vi "Default Property or Method.vi"(8 "error in":errorcluster, 10 "Properties for Tree In":T1(array[cluster]), 11 "Affected Items":T2) -> (0 "error out":errorcluster, 3 "One default element":bool)   [LabVIEW 2023]
doc: "Determine if the property or invoke node contains only the default property (such as when the node is first dropped)."
uses:
  top/BundleMagic.ctl
panel:
  # "Take either input"
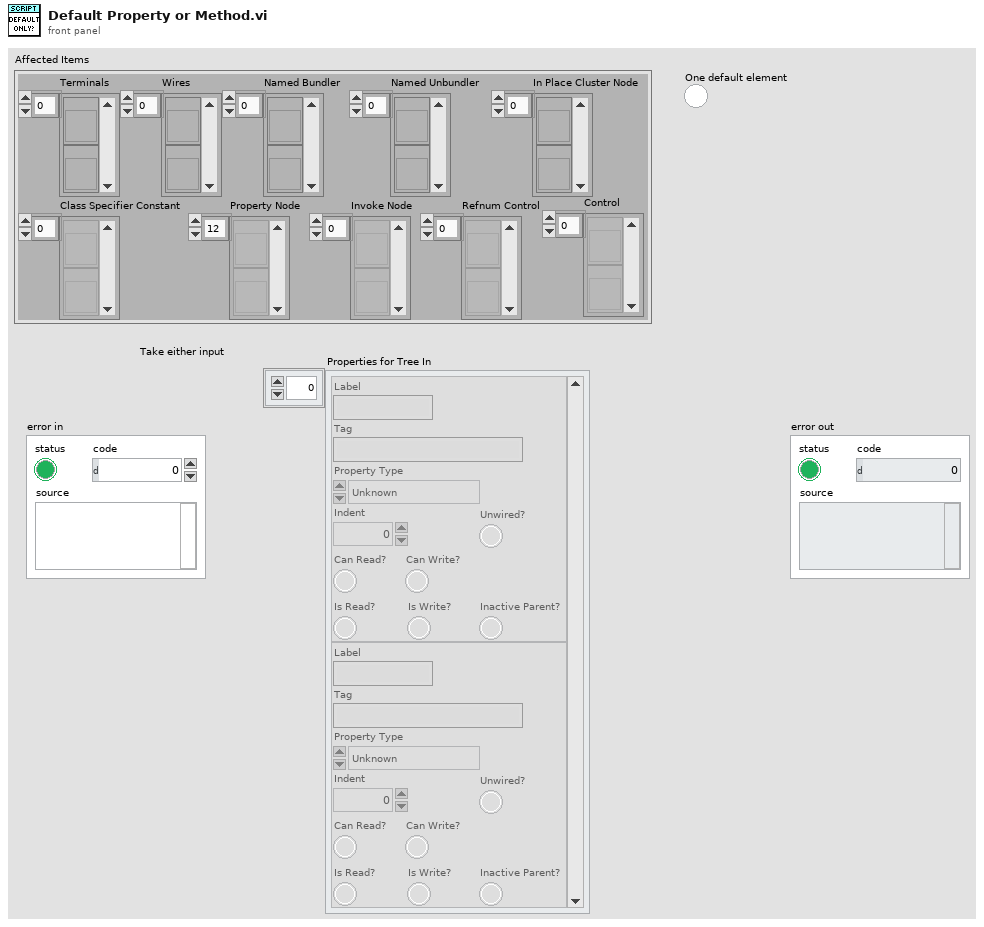
[diagram p1: front panel]
types:
  T1 = cluster{"Label":string, "Tag":string, "Property Type":enum16{"Unknown", "Base", "Scripting", "Private", "Deprecated", "None", "Divider"}, "Indent":u16, "Can Read?":bool, "Can Write?":bool, "Is Read?":bool, "Is Write?":bool, "Inactive Parent?":bool, "Unwired?":bool}[]
  T2 = typedef "BundleMagic.ctl" = cluster{"Terminals":refnum<vi>[], "Wires":refnum<vi>[], "Named Bundler":refnum<vi>[], "Named Unbundler":refnum<vi>[], "In Place Cluster Node":refnum<vi>[], "Class Specifier Constant":refnum<vi>[], "Property Node":refnum<vi>[], "Invoke Node":refnum<vi>[], "Refnum Control":refnum<vi>[], "Control":refnum<vi>[]}
  T3 = cluster{"Label":string, "Tag":string, "Property Type":enum16{"Unknown", "Base", "Scripting", "Private", "Deprecated", "None", "Divider"}, "Indent":u16, "Can Read?":bool, "Can Write?":bool, "Is Read?":bool, "Is Write?":bool, "Inactive Parent?":bool, "Unwired?":bool}
  T4 = typedef "ASPM_UniqueIDStringDatanameShortnameLongname.ctl" = cluster{"Unique ID string":string, "Data name":string, "Short name (localized)":string, "Long name (localized)":string}
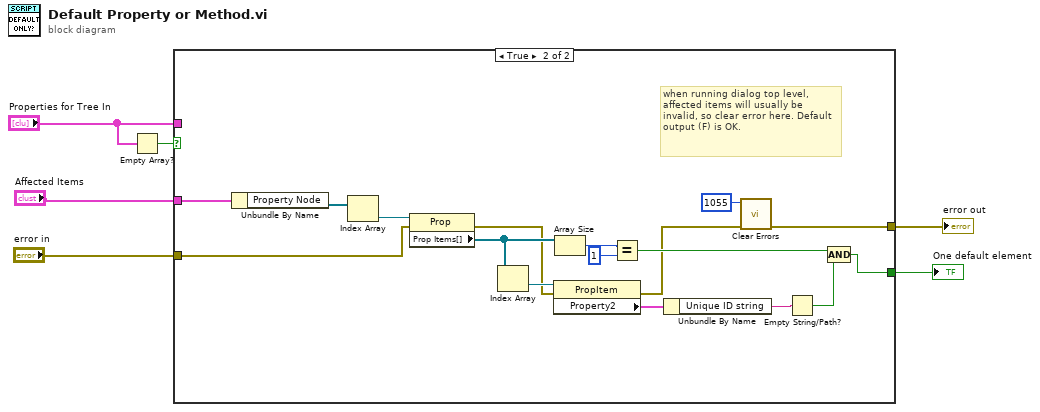
[diagram p0: block diagram]
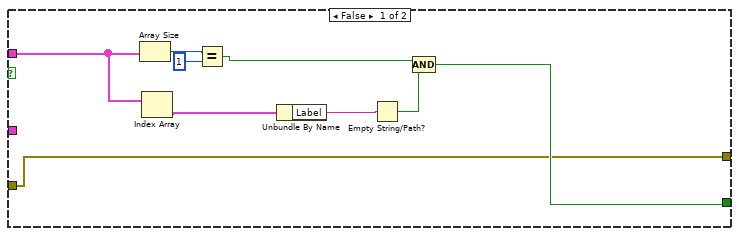
[diagram p2: hidden frame]
diagram:
  n1 = Empty Array?(array="Properties for Tree In") -> (empty?=w2:bool)
  n2 = case shown="True" w2 {
    tunnel: "Affected Items" -> [_ w31]
    tunnel: "error in" -> [w7 w30]
    tunnel: [w7 w17] -> w4
    tunnel: [w8 w29] -> w3
    tunnel: "Properties for Tree In" -> [w10 _]
    frame False {
      n3 = Array Size(array=w10) -> (size(s)=w15:i32)
      n4 = Index Array(array=w10) -> (element=w9:T3)  [unwired: 1 in]
      n5 = Equal?(x=w15, y=1) -> (x = y?=w14:bool)
      n6 = Unbundle By Name(w9) -> ("Label"=w13:string)
      n7 = Empty String/Path?(string/path=w13) -> (empty?=w12:bool)
      n8 = Compound Arithmetic op=AND(w14, w12) -> (w8:bool)
    }
    frame True {
      # "when running dialog top level, affected items will usually be invalid, so clear error here. Default output (F) is OK."
      n9 = Unbundle By Name(w31) -> ("Property Node"=w28:refnum<vi>[])
      n10 = Index Array(array=w28) -> (element=w32:refnum<vi>)  [unwired: 1 in]
      n11 = property class="Prop"(reference=w32, error in=w30) -> (error out=w19:errorcluster, "Prop Items[]"=w24:refnum<vi>[])  [unwired: 1 out]
      n12 = Index Array(array=w24) -> (element=w27:refnum<vi>)  [unwired: 1 in]
      n13 = property class="PropItem"(reference=w27, error in=w19) -> (error out=w18:errorcluster, "Property2"=w22:T4)  [unwired: 1 out]
      n14 = Array Size(array=w24) -> (size(s)=w26:i32)
      n15 = Equal?(x=w26, y=1) -> (x = y?=w23:bool)
      n16 = Unbundle By Name(w22) -> ("Unique ID string"=w21:string)
      n17 = call <vilib>:"Clear Errors.vi"("error in (no error)"=w18, "specific error code to clear (0: all)"=1055) -> ("error out"=w17:errorcluster)  [unwired: 4 in, 1 out]
      n18 = Empty String/Path?(string/path=w21) -> (empty?=w20:bool)
      n19 = Compound Arithmetic op=AND(w23, w20) -> (w29:bool)
    }
  }
  "error out" <- w4
  "One default element" <- w3
